vi "SelectTemplate.vi"() -> (0 "Success":bool, 1 "name":string)   [LabVIEW 2012]
panel:
  in  "Tab Control":enum32{"Templ", "name"}(tab)
  in  "Available Templates":i32(listbox)
  in  "Ok":bool
  in  "Cancel":bool
  in  "Name":string
  in  "Cancel 2":bool
  in  "Ok 2":bool
  # "Enter a silde name"
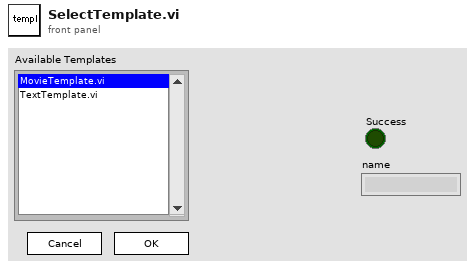
[diagram p1: front panel]
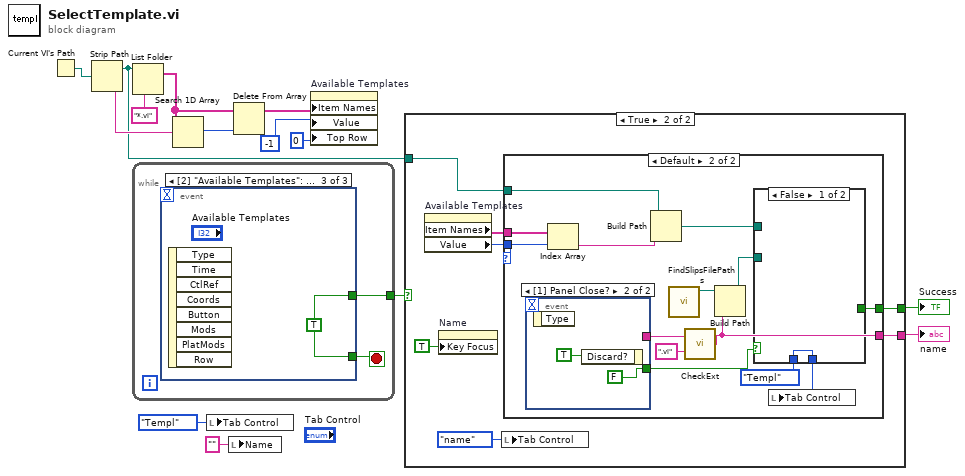
[diagram p0: block diagram]
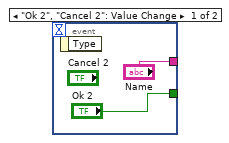
[diagram p4: hidden frame]
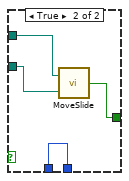
[diagram p5: hidden frame]
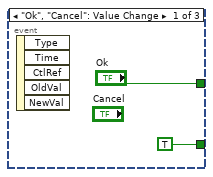
[diagram p6: hidden frame]
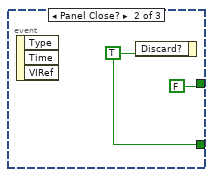
[diagram p7: hidden frame]
diagram:
  n1 = Current VI's Path() -> (path=w13:path)
  n2 = Strip Path(path=w13) -> (stripped path=w6:path, name=w12:string)
  n3 = List Folder(path=w6, pattern="*.vi") -> (filenames=w10:string[])  [unwired: 2 in, 3 out]
  n4 = while {
    tunnel: [w15] -> w7
    stop <- w16 stop-if-true
    n5 = event shown="[2] \"Available Templates\": Double Click" {
      selector: _ -> [_ _ _]
      dyn-events: _ -> [_ _ _]
      timeout: _ -> [_ _ _]
      tunnel: [TRUE w20 w21] -> w16
      tunnel: ["Ok" FALSE w21] -> w15
      event "Ok", "Cancel": Value Change {
        n6 = event-data() -> ()  [unwired: 1 in, 5 out]
      }
      event Panel Close? {
        w20 = TRUE
        n7 = event-data() -> ()  [unwired: 1 in, 3 out]
        n8 = event-data("Discard?"=w20) -> ()  [unwired: 1 in, 1 out]
      }
      event "Available Templates": Double Click {
        w21 = TRUE
        n9 = event-data() -> ()  [unwired: 1 in, 8 out]
      }
    }
  }
  n10 = Search 1D Array(1D array=w10, element=w12) -> (index of element=w11:i32)  [unwired: 1 in]
  n11 = local write "Tab Control"(enum32{"Templ", "name"}."Templ" ("Tab Control")) -> ()
  n12 = local write "Name"("" ("Name")) -> ()
  n13 = Delete From Array(array=w10, index=w11) -> (array with subset deleted=w9:string[])  [unwired: 1 in, 1 out]
  n14 = property on="Available Templates" class="LstBox (strict)"("Item Names"=w9, "Value"=-1 ("Available Templates"), "Top Row"=0 ("Available Templates")) -> ()  [unwired: 2 in, 2 out]
  n15 = case shown="True" w7 {
    tunnel: w6 -> [_ w27]
    tunnel: [_ w25] -> w5
    tunnel: [_ w24] -> w4
    frame False {
    }
    frame True {
      n16 = property on="Available Templates" class="LstBox (strict)"() -> ("Item Names"=w28:string[], "Value"=w26:i32)  [unwired: 2 in, 2 out]
      n17 = property on="Name" class="Str"("Key Focus"=TRUE) -> ()  [unwired: 2 in, 2 out]
      n18 = local write "Tab Control"(enum32{"Templ", "name"}."name" ("Tab Control")) -> ()
      n19 = case shown="Default" w26 {
        tunnel: w28 -> [_ w42]
        tunnel: w27 -> [_ w41]
        tunnel: w26 -> [_ w39]
        tunnel: [_ w36] -> w25
        tunnel: [_ w32] -> w24
        frame -1 {
        }
        frame Default {
          n20 = event shown="[1] Panel Close?" {
            selector: _ -> [_ _]
            dyn-events: _ -> [_ _]
            timeout: _ -> [_ _]
            tunnel: ["Name" _] -> w33
            tunnel: ["Ok 2" FALSE] -> w35
            event "Ok 2", "Cancel 2": Value Change {
              n21 = event-data() -> ()  [unwired: 1 in, 1 out]
            }
            event Panel Close? {
              n22 = event-data() -> ()  [unwired: 1 in, 1 out]
              n23 = event-data("Discard?"=TRUE) -> ()  [unwired: 1 in, 1 out]
            }
          }
          n24 = Index Array(array=w42, index=w39) -> (element=w31:string)
          n25 = Build Path(base path=w41, name or relative path=w31) -> (appended path=w40:path)
          n26 = call "FindSlipsFilePaths.vi"() -> ("Slides"=w38:path)  [unwired: 2 in, 4 out]
          n27 = call "CheckExt.vi"("extension"=".vi" ("search string/char (-)"), "Name in"=w33) -> ("Name"=w32:string)
          n28 = Build Path(base path=w38, name or relative path=w32) -> (appended path=w37:path)
          n29 = case shown="False" w35 {
            tunnel: w40 -> [_ w51]
            tunnel: w37 -> [_ w50]
            tunnel: [_ w49] -> w36
            tunnel: [w47 w48] -> w30
            tunnel: enum32{"Templ", "name"}."Templ" ("Tab Control") -> [w47 w48]
            frame False {
            }
            frame True {
              n30 = call "MoveSlide.vi"("Target"=w50, "Source"=w51) -> ("Success?"=w49:bool)
            }
          }
          n31 = local write "Tab Control"(w30) -> ()
        }
      }
    }
  }
  "Success" <- w5
  "name" <- w4
